vi "Create Log File.vi"(8 "error in (no error)":errorcluster, 11 "EventRecorder in":refnum<class "EventRecorder.lvclass">) -> (0 "error out":errorcluster, 3 "EventRecorder out":refnum<class "EventRecorder.lvclass">)   [LabVIEW 2019, in "EventRecorder.lvlib" / "EventRecorder.lvclass"]
uses:
  EventRecorder.lvclass
  EventRecorder.lvclass/EventRecorder.ctl
  <vilib>/NI/Event Logger Library/EventLog/Initialize_CSV.vi
  <vilib>/NI/Event Logger Library/EventLog/EventLog.lvclass
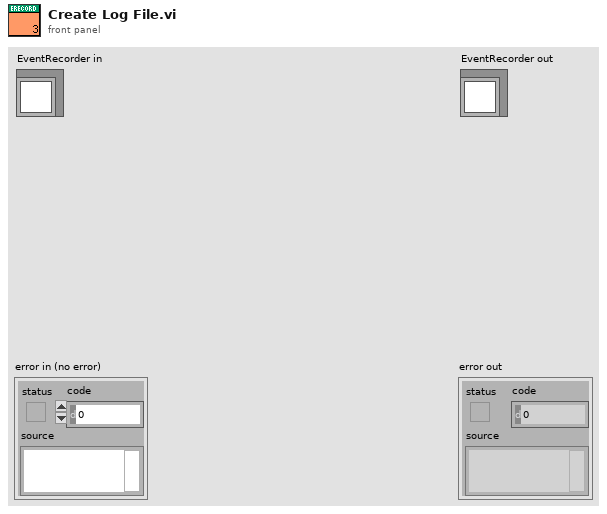
[diagram p1: front panel]
types:
  T1 = enum16{"open", "replace", "create", "open or create", "replace or create", "replace or create with confirmation"}
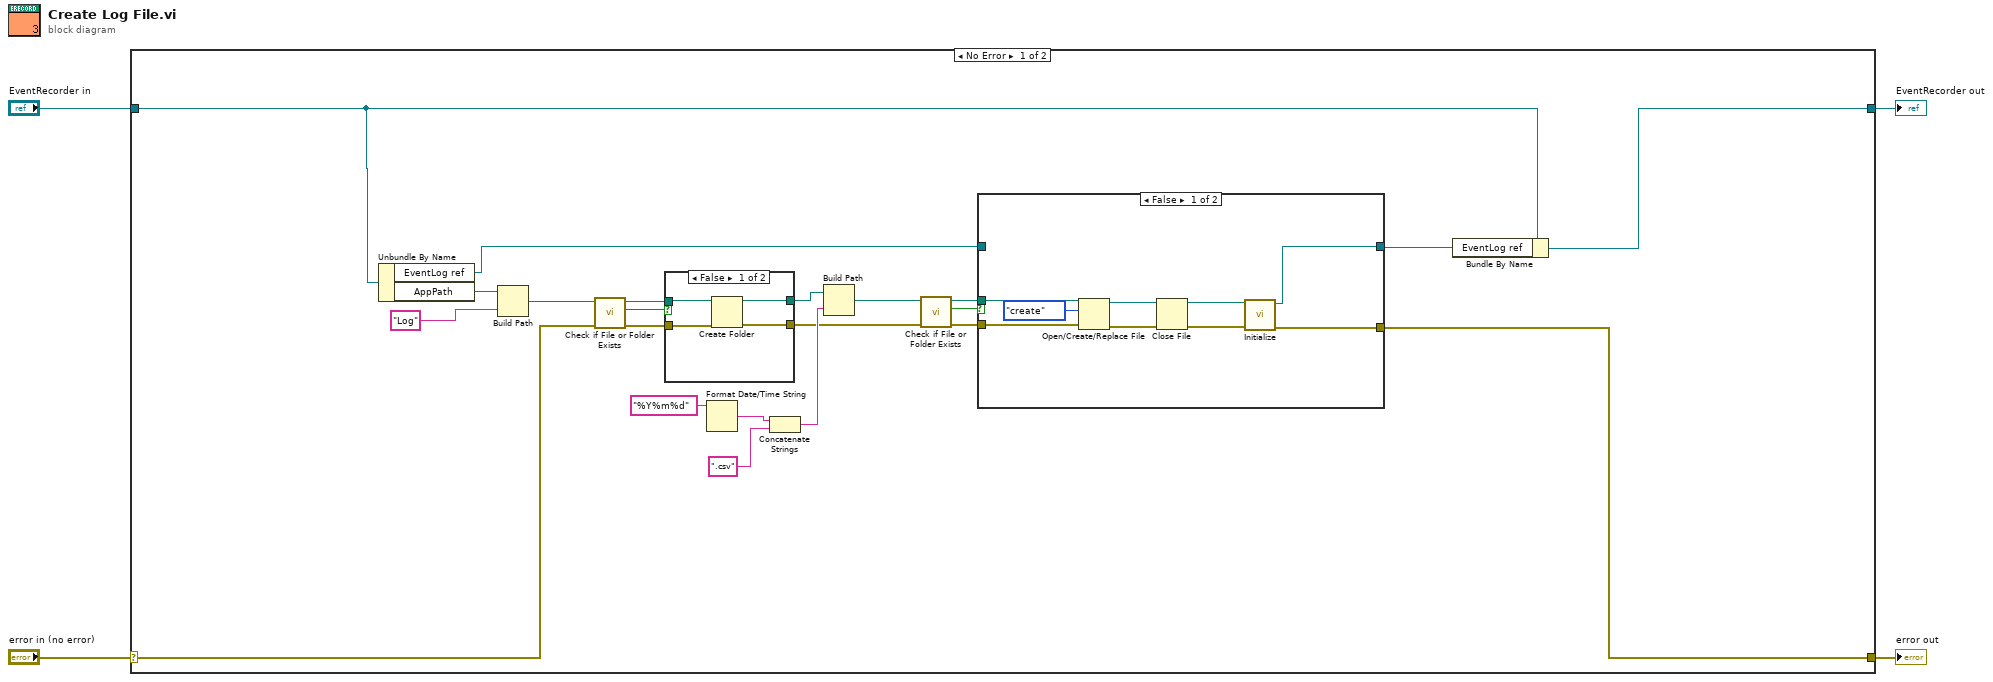
[diagram p0: block diagram]
diagram:
  n1 = case shown="No Error" "error in (no error)" {
    selector: "error in (no error)" -> [w6 w45]
    tunnel: [w5 w45] -> w3
    tunnel: [w7 w44] -> w1
    tunnel: "EventRecorder in" -> [w8 w44]
    frame No Error {
      n2 = Unbundle By Name(w8) -> ("EventLog ref"=w10:refnum<class "EventLog.lvclass">, "AppPath"=w26:path)
      n3 = Build Path(base path=w26, name or relative path="Log") -> (appended path=w21:path)
      n4 = call <vilib>:"Check if File or Folder Exists.vi"("error in (no error)"=w6, "path"=w21) -> ("error out"=w12:errorcluster, "file or folder exists?"=w20:bool, "dup path"=w19:path)  [unwired: 7 in]
      n5 = case shown="False" w20 {
        tunnel: w19 -> [w41 w43]
        tunnel: [w40 w43] -> w18
        tunnel: w12 -> [w39 w42]
        tunnel: [w38 w42] -> w11
        frame False {
          n6 = Create Folder(path (use dialog)=w41, error in=w39) -> (created path=w40:path, error out=w38:errorcluster)  [unwired: 1 in, 1 out]
        }
        frame True {
        }
      }
      n7 = Format Date/Time String(time format string (%c)="%Y%m%d") -> (date/time string=w23:string)  [unwired: 2 in]
      n8 = Concatenate Strings(w23, ".csv" ("string")) -> (w17:string)
      n9 = Build Path(base path=w18, name or relative path=w17) -> (appended path=w16:path)
      n10 = call <vilib>:"Check if File or Folder Exists.vi"("error in (no error)"=w11, "path"=w16) -> ("error out"=w13:errorcluster, "file or folder exists?"=w15:bool, "dup path"=w14:path)  [unwired: 7 in]
      n11 = case shown="False" w15 {
        tunnel: w14 -> [w35 _]
        tunnel: w13 -> [w31 w37]
        tunnel: [w28 w37] -> w5
        tunnel: w10 -> [_ w36]
        tunnel: [w27 w36] -> w9
        frame False {
          n12 = Open/Create/Replace File(file path (use dialog)=w35, error in=w31, operation (0:open)=T1."create") -> (refnum out=w33:refnum<file>, error out=w32:errorcluster)  [unwired: 3 in, 1 out]
          n13 = Close File(refnum=w33, error in=w32) -> (path=w30:path, error out=w29:errorcluster)
          n14 = call-poly <vilib>:"Initialize.vi"("error in (no error)"=w29, "Path"=w30) -> ("error out"=w28:errorcluster, "EventLog ref"=w27:refnum<class "EventLog.lvclass">)  [unwired: 8 in]
        }
        frame True {
        }
      }
      n15 = Bundle By Name(cluster=w8, "EventLog ref"=w9) -> (w7:refnum<class "EventRecorder.lvclass">)
    }
    frame Error {
    }
  }
  "error out" <- w3
  "EventRecorder out" <- w1
